vi "String - Convert MessageCode and Remarks to [ColumnData].vi"(11 "<. ....> + Pre-Description<PrePost>Post-Description":string) -> (0 "Message Code <.....> Found":bool, 1 "[MessageId]":string, 2 "[MessageType]":string, 3 "PrePost Description":cluster{"Pre":string, "Post":string}, 4 "<NoML>":bool, 5 "<. ....>":string, 6 "<NoD>":bool)   [LabVIEW 2020]
panel:
  out "Pre-Description<PrePost>Post-Description":string
  # "<I 123>Hello<PrePost>World"
  # "Customer Name: A25B 3762 0D54 F079"
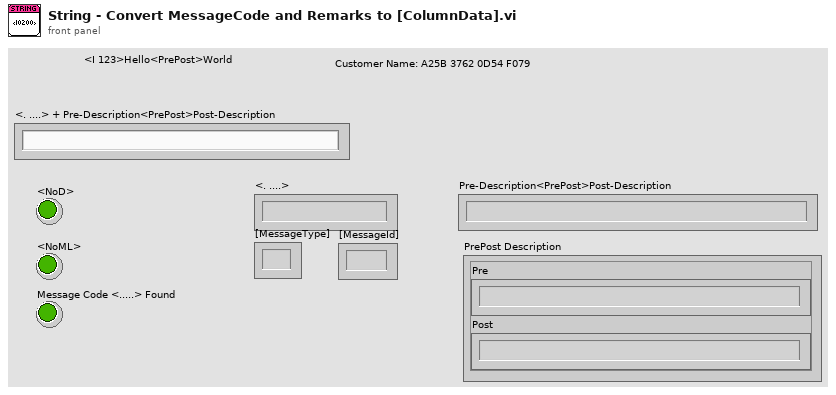
[diagram p1: front panel]
types:
  T1 = cluster{"result string":string, "result string":string}
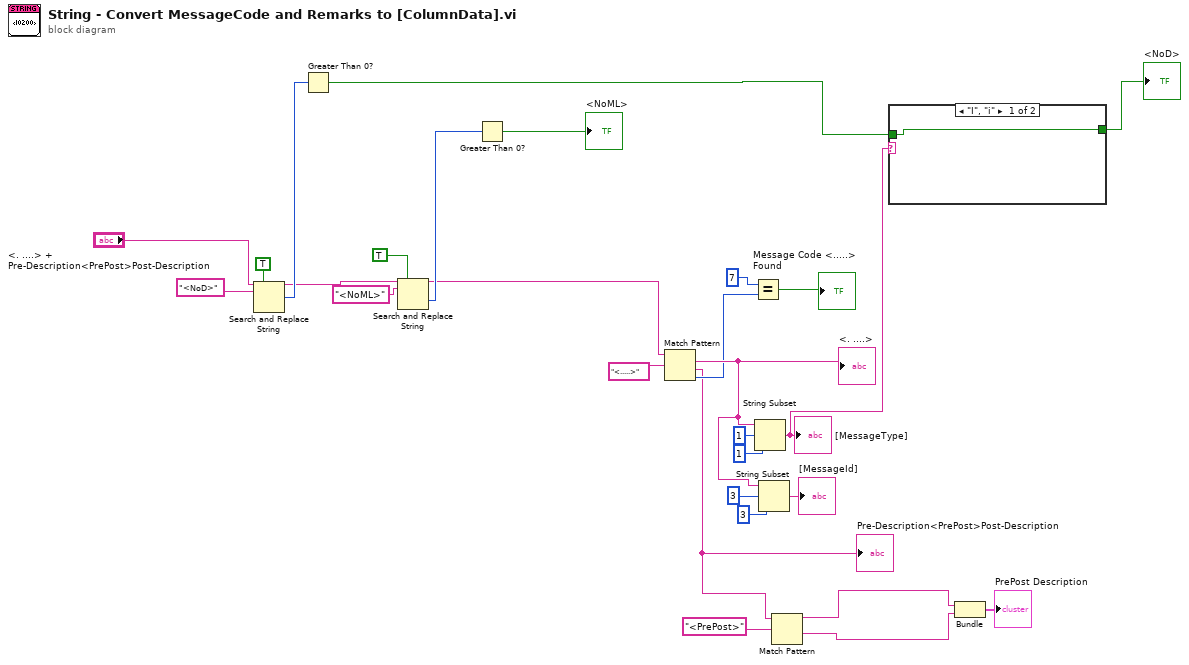
[diagram p0: block diagram]
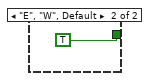
[diagram p2: hidden frame]
diagram:
  n1 = Search and Replace String(replace all?=TRUE ("replace all? (F)"), input string="<. ....> + Pre-Description<PrePost>Post-Description", search string="<NoD>") -> (result string=w15:string, number of replacements=w17:i32)  [unwired: 5 in, 2 out]
  n2 = Greater Than 0?(x=w17) -> (x > 0?=w2:bool)
  n3 = Search and Replace String(replace all?=TRUE ("replace all? (F)"), input string=w15, search string="<NoML>") -> (result string=w10:string, offset past replacement=w12:i32)  [unwired: 5 in, 2 out]
  n4 = Greater Than 0?(x=w12) -> (x > 0?=→"<NoML>":bool)
  n5 = Match Pattern(string=w10, regular expression="<.....>") -> (match substring=w22:string, after substring=w8:string, offset past match=w21:i32)  [unwired: 1 in, 1 out]
  "<. ....>" <- w22
  "Pre-Description<PrePost>Post-Description" <- w8
  n6 = Equal?(x=7, y=w21) -> (x = y?=→"Message Code <.....> Found":bool)
  n7 = String Subset(string=w22, offset (0)=1, length (rest)=1 ("length (rest)")) -> (substring=w3:string)
  "[MessageType]" <- w3
  n8 = String Subset(string=w22, offset (0)=3, length (rest)=3 ("length (rest)")) -> (substring=→"[MessageId]":string)
  n9 = Match Pattern(string=w8, regular expression="<PrePost>") -> (before substring=w6:string, after substring=w5:string)  [unwired: 1 in, 2 out]
  n10 = case shown="\"I\", \"i\"" w3 {
    tunnel: w2 -> [w29 _]
    tunnel: [w29 TRUE] -> w1
    frame "I", "i" {
    }
    frame "E", "W", Default {
    }
  }
  "<NoD>" <- w1
  n11 = Bundle("result string"=w6, "result string"=w5) -> (→"PrePost Description":T1)  [unwired: 1 in]
